vi "Fetch Measurement (Single Point).vi"(0 "VISA resource name":refnum<visa-resource-name>, 11 "error in (no error)":errorcluster) -> (3 "Go":bool, 4 "VISA resource name out":refnum<visa-resource-name>, 6 "Measurement":dbl, 10 "Questionable Data":bool, 13 "High":bool, 14 "Low":bool, 15 "error out":errorcluster)   [LabVIEW 2017, in "ADCMT 6240.lvlib"]
doc: "Fetches and returns a single measurement from the instrument."
uses:
  ADCMT 6240.lvlib
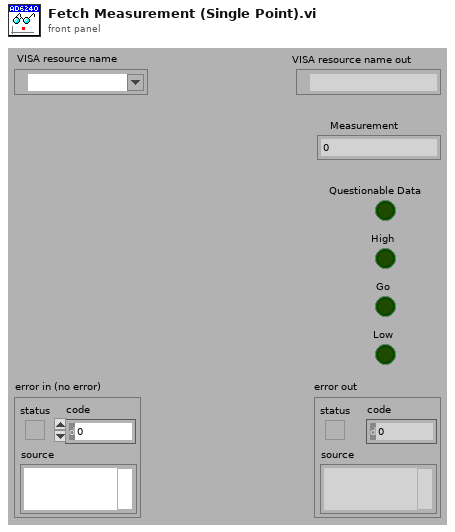
[diagram p1: front panel]
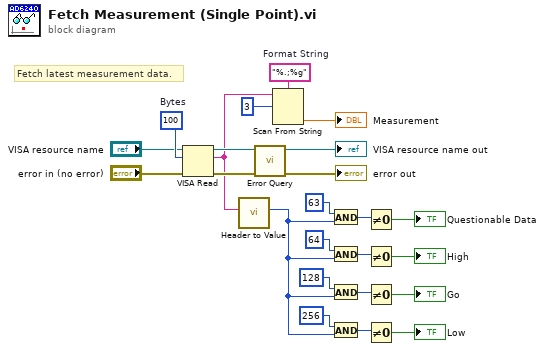
[diagram p0: block diagram]
diagram:
  w23 = "%.;%g"  # Format String
  w24 = u32 100  # Bytes
  # "Fetch latest measurement data."
  n1 = VISA Read ("VISA読み取り")(VISA resource name="VISA resource name", byte count=w24, error in (no error)="error in (no error)") -> (VISA resource name out=w18:refnum<visa-resource-name>, read buffer=w15:string, error out=w21:errorcluster)  [unwired: 1 out]
  n2 = call "Header to Value.vi"("Header String (\"\")"=w15) -> ("Header Information"=w5:u32)  [unwired: 10 in]
  n3 = call "Error Query.vi"("error in (no error)"=w21, "VISA resource name"=w18) -> ("error out"=→"error out":errorcluster, "VISA resource name out"=→"VISA resource name out":refnum<visa-resource-name>)  [unwired: 6 in, 2 out]
  n4 = Scan From String ("文字列からスキャン")(format string=w23, input string=w15, initial scan location=3) -> (output 1=→"Measurement":dbl)  [unwired: 2 in, 3 out]
  n5 = And(x=63, y=w5) -> (x .and. y?=w12:u32)
  n6 = And(x=64, y=w5) -> (x .and. y?=w11:u32)
  n7 = And(x=128, y=w5) -> (x .and. y?=w8:u32)
  n8 = And(x=256, y=w5) -> (x .and. y?=w7:u32)
  n9 = Not Equal To 0?(x=w12) -> (x != 0?=→"Questionable Data":bool)
  n10 = Not Equal To 0?(x=w11) -> (x != 0?=→"High":bool)
  n11 = Not Equal To 0?(x=w8) -> (x != 0?=→"Go":bool)
  n12 = Not Equal To 0?(x=w7) -> (x != 0?=→"Low":bool)
